vi "Reset.vi"(8 "error in":errorcluster, 11 "9115AT in":refnum<class "9115AT.lvclass">) -> (0 "error out":errorcluster, 3 "9115AT out":refnum<class "9115AT.lvclass">)   [LabVIEW 2018, in "9115AT.lvlib" / "9115AT.lvclass"]
uses:
  9115AT.lvclass
  <instrlib>/BK Precision 911X Series/BK Precision 911X Series.lvlib
  builds/Power_Supply.lvlibp/Power Supply.lvclass
  C:/Users/Ron.Dexter.LUMINARTECH/Desktop/builds/Power_Supply.lvlibp/Power Supply.lvclass
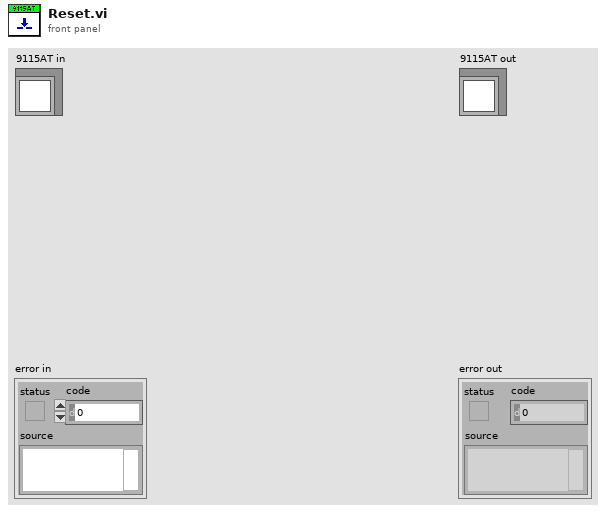
[diagram p1: front panel]
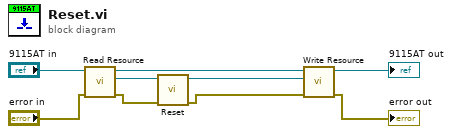
[diagram p0: block diagram]
diagram:
  n1 = call "Read Resource.vi"("error in"="error in", "Power Supply in"="9115AT in") -> ("error out"=w3:errorcluster, "Resource"=w7:refnum<visa-resource-name>, "Power Supply out"=w5:refnum<class "9115AT.lvclass">)  [unwired: 7 in]
  n2 = call <instrlib>:"Reset.vi"("error in (no error)"=w3, "VISA resource name"=w7) -> ("error out"=w2:errorcluster, "VISA resource name out"=w6:refnum<visa-resource-name>)  [unwired: 8 in]
  n3 = call "Write Resource.vi"("error in"=w2, "Resource"=w6, "Power Supply in"=w5) -> ("error out"=→"error out":errorcluster, "Power Supply out"=→"9115AT out":refnum<class "9115AT.lvclass">)  [unwired: 7 in]
